vi "Set Video Mode.vi"(8 "error in (no error)":errorcluster, 9 "Video Line Marker (1)":i32=1, 10 "Video Format (0: NTSC)":u32(ring) items=["NTSC", "PAL", "PALM (for PAL-M)", "SECAM"], 11 "VISA resource name":refnum<visa-resource-name>) -> (0 "error out":errorcluster, 3 "VISA resource name out":refnum<visa-resource-name>)   [LabVIEW 2014, in "Fluke 5XXX Series Multicalibrators.lvlib"]
doc: "This VI selects the format for Video scope mode and programs the Video mode line marker location.\n\nNote:\n\nThis VI is available only for instrument models 5500A and 5520A with oscilloscope option SC600 (SC1100)."
uses:
  Fluke 5XXX Series Multicalibrators.lvlib
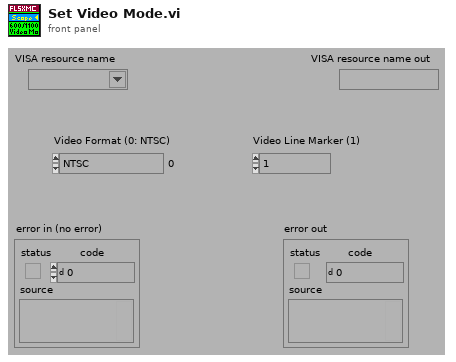
[diagram p1: front panel]
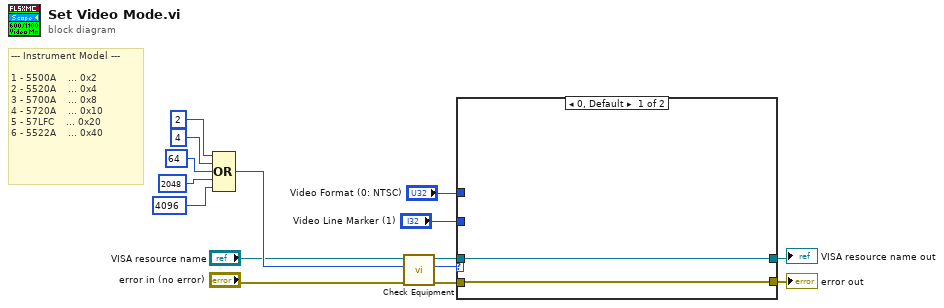
[diagram p0: block diagram]
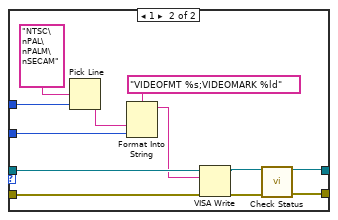
[diagram p2: hidden frame]
diagram:
  # "--- Instrument Model ---\n\n1 - 5500A    ... 0x2\n2 - 5520A    ... 0x4\n3 - 5700A    ... 0x8\n4 - 5720A    ... 0x10\n5 - 57LFC    ... 0x20\n6 - 5522A    ... 0x40"
  n1 = Compound Arithmetic op=OR(2 ("Numeric"), 4 ("Numeric"), 64 ("Numeric"), 2048 ("Numeric"), 4096 ("Numeric")) -> (w9:i32)
  n2 = call "Check Equipment.vi"("error in (no error)"="error in (no error)", "Bit Mask"=w9, "VISA resource name"="VISA resource name") -> ("error out"=w12:errorcluster, "Present?"=w11:u32, "VISA resource name out"=w10:refnum<visa-resource-name>)  [unwired: 6 in]
  n3 = case shown="0, Default" w11 {
    tunnel: [w16 w23] -> w4
    tunnel: w12 -> [w17 w28]
    tunnel: w10 -> [w16 w27]
    tunnel: [w17 w26] -> w5
    tunnel: "Video Line Marker (1)" -> [_ w19]
    tunnel: "Video Format (0: NTSC)" -> [_ w18]
    frame 0, Default {
    }
    frame 1 {
      n4 = Pick Line(multi-line string="NTSC\nPAL\nPALM\nSECAM", line index=w18) -> (output string=w22:string)  [unwired: 1 in]
      n5 = Format Into String(format string="VIDEOFMT %s;VIDEOMARK %ld" ("Reset Command"), w22, w19) -> (resulting string=w20:string)  [unwired: 2 in, 1 out]
      n6 = VISA Write(VISA resource name=w27, write buffer=w20, error in (no error)=w28) -> (VISA resource name out=w24:refnum<visa-resource-name>, error out=w25:errorcluster)  [unwired: 1 out]
      n7 = call "Check Status.vi"("VISA resource name"=w24, "error in (no error)"=w25) -> ("VISA resource name out"=w23:refnum<visa-resource-name>, "error out"=w26:errorcluster)  [unwired: 12 in]
    }
  }
  "VISA resource name out" <- w4
  "error out" <- w5
